vi "Move XY Raster.vi"(4 "Initial Y Direction":bool=TRUE, 6 "Initial X Direction":bool=TRUE, 8 "Error In":errorcluster, 9 "Y Number of Steps":string="0", 10 "X Number of Steps":string="0", 11 "Reference In":refnum<class "_Controller.lvclass">) -> (0 "Error Out":errorcluster, 3 "Reference Out":refnum<class "_Controller.lvclass">)   [LabVIEW 2020]
doc: "Bi-axial raster scan logic for the XY plane. Performs the uni-axial raster scan logic in the X direction then moves along 1 scanning point in the Y dirction. This is the looped to cover the entire area.\n\nArgs:\n\nReference In: Incoming communication (reference) between LabView and the scanning rig controller\nX Number of Steps: Total number of steps to move along that axis\nY Number of Steps: Total number of steps to move along that axis\nInitial X Direction: Initial X direction for the scan\nInitial Y Direction: Initial Y direction for the scan\nError In: Checks for any errors with the incoming communication (reference)\n\nReturns:\n\nReference Out: Output communnication (reference) between LabView and controller\nError Out: Checks for any error with output communication (reference)"
uses:
  <instrlib>/Arcus Ethernet Driver 1.0.0/ArcusEthernetComm/classes/Controller/_Controller.lvclass
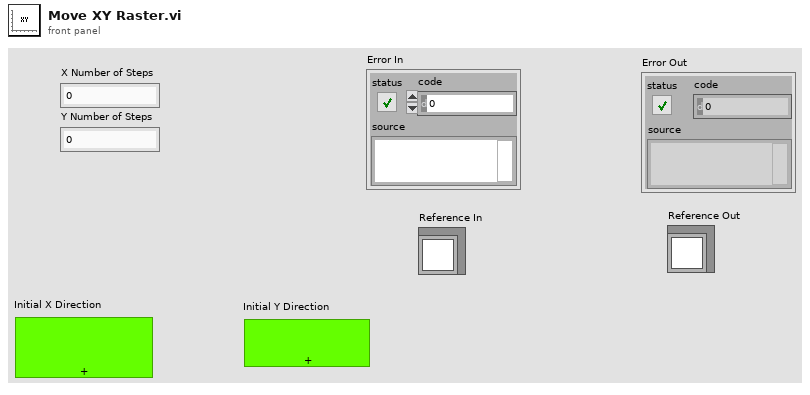
[diagram p1: front panel]
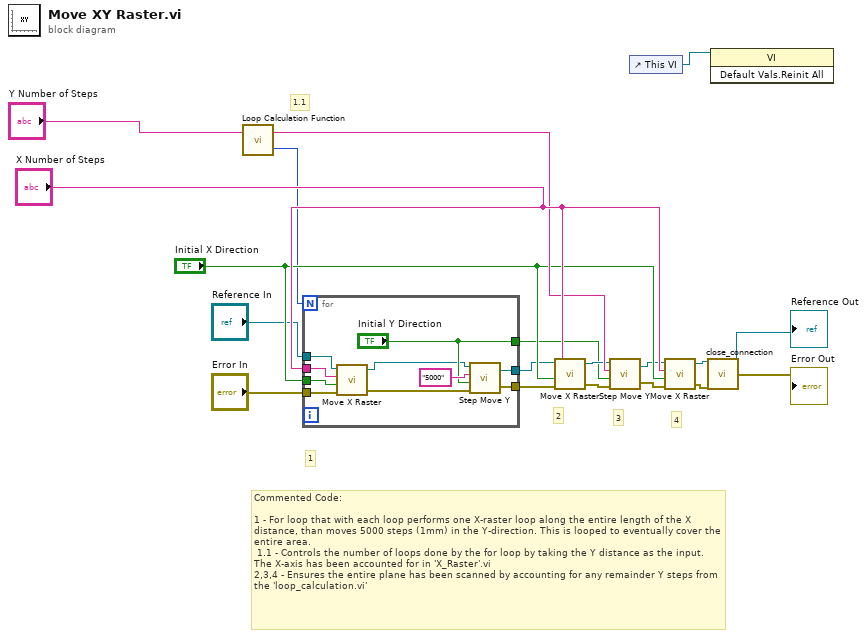
[diagram p0: block diagram]
diagram:
  # "Commented Code:\n\n1 - For loop that with each loop performs one X-raster loop along the entire length of the X distance, than moves 5000 steps (1mm) in the Y-direction. This is looped to eventually cover the entire area.\n 1.1 - Controls the number of loops done by the for loop by taking the Y distance as the input. The X-axis has been accounted for in 'X_Raster'.vi\n2,3,4 - Ensures the entire plane has been scanned by accounting for any remainder Y steps from the 'loop_calculation.vi'"
  # "4"
  # "3"
  # "2"
  # "1.1"
  # "1"
  n1 = call "Loop Calculation Function.vi"("Number of Steps"="Y Number of Steps") -> ("No. of Scan Points"=w3:i32, "Remainder"=w18:string)  [unwired: 1 in]
  n2 = for {
    N: w3 -> [_]
    tunnel: "X Number of Steps" -> [w27]
    tunnel: "Initial X Direction" -> [w28]
    tunnel: ["Initial Y Direction"] -> w7
    tunnel: [w24] -> w6
    tunnel: [w23] -> w5
    tunnel: "Reference In" -> [w21]
    tunnel: "Error In" -> [w20]
    n3 = call "Move X Raster.vi"("Error In"=w20, "Initial Direction"=w28, "X Number of Steps"=w27, "Reference In"=w21) -> ("Error Out"=w22:errorcluster, "Reference Out"=w25:refnum<class "_Controller.lvclass">)  [unwired: 1 in]
    n4 = call "Step Move Y.vi"("Error In"=w22, "Direction"="Initial Y Direction", "No. of Y Steps"="5000" ("Y Steps"), "Reference In"=w25) -> ("Error Out"=w23:errorcluster, "Reference Out"=w24:refnum<class "_Controller.lvclass">)
  }
  n5 = call "Move X Raster.vi"("Error In"=w5, "Initial Direction"="Initial X Direction", "X Number of Steps"="X Number of Steps", "Reference In"=w6) -> ("Error Out"=w13:errorcluster, "Reference Out"=w14:refnum<class "_Controller.lvclass">)  [unwired: 1 in]
  n6 = call "Step Move Y.vi"("Error In"=w13, "Direction"=w7, "No. of Y Steps"=w18, "Reference In"=w14) -> ("Error Out"=w12:errorcluster, "Reference Out"=w11:refnum<class "_Controller.lvclass">)
  n7 = control-ref of="This VI"() -> (w2:refnum<vi>)
  n8 = call "Move X Raster.vi"("Error In"=w12, "Initial Direction"="Initial X Direction", "X Number of Steps"="X Number of Steps", "Reference In"=w11) -> ("Error Out"=w16:errorcluster, "Reference Out"=w17:refnum<class "_Controller.lvclass">)  [unwired: 1 in]
  n9 = call <instrlib>:"close_connection.vi"("reference (in)"=w17, "error in (no error)"=w16) -> ("reference (out)"=→"Reference Out":refnum<class "_Controller.lvclass">, "error out"=→"Error Out":errorcluster)  [unwired: 16 in]
  n10 = invoke class="VI" method="Default Vals.Reinit All"(reference=w2) -> ()  [unwired: 2 in, 3 out]
